vi "Start.vi"(8 "error in (no error)":errorcluster, 11 "Framework in":refnum<class "Framework.lvclass">) -> (0 "error out":errorcluster, 3 "Framework out":refnum<class "Framework.lvclass">)   [LabVIEW 2019, in "DSF Core.lvlib" / "Framework.lvclass"]
uses:
  Framework.lvclass
  Framework States.ctl
  Framework.lvclass/Framework.ctl
  <vilib>/NI/Memory Manager/Classes/Pointer/Pointer.lvclass/Pointer.ctl
  Interface/Interface.lvclass/Interface.ctl
  Pointers/Error/Error Pointer.lvclass/Error Pointer.ctl
  Interface/Dispatcher/Write.vi
  Interface/Dispatcher/Write Dispatcher Command.vi
  Interface/Errors.vi
  Interface/Dispatcher/Invalid Response.vi
  Interface/Dispatcher/Read.vi
  Interface/Dispatcher/Read Dispatcher Response.vi
  Interface/Logging/Send.vi
  Interface/Logging/Send Logging Command.vi
  Interface/Logging/Wait For.vi
  Interface/Logging/Wait For Logging Response.vi
  <vilib>/NI/Memory Manager/Classes/Pointer/Write.vi
  <vilib>/NI/Memory Manager/Classes/Pointer/Write U8.vi
  Read State.vi
  Pointers/Error/Write Error Pointer.vi
  <vilib>/NI/Memory Manager/Classes/Pointer/Get Address.vi
  Interface/Send Command.vi
  Interface/Dispatcher/Command Timeout.vi
  Interface/Dispatcher/Class Name.vi
  <vilib>/NI/Memory Manager/VIs/Write String to Source.vi
  Interface/New Interface Error.vi
  Interface/Wait For Response.vi
  Interface/Dispatcher/Response Timeout.vi
  <vilib>/NI/Memory Manager/Classes/Pointer/Write (No Check).vi
  <vilib>/NI/Memory Manager/Classes/Pointer/Write (No Check) U8.vi
  <vilib>/NI/Memory Manager/Classes/Pointer/Check Move.vi
  <vilib>/NI/Memory Manager/Classes/Pointer/Read.vi
  <vilib>/NI/Memory Manager/Classes/Pointer/Read U8.vi
  <vilib>/NI/Memory Manager/Classes/Pointer/Write 1D U8.vi
  <vilib>/NI/Memory Manager/Classes/Pointer/Clear.vi
  Pointers/Error/Get Power Of 2.vi
  Interface/Write RT FIFO.vi
  <vilib>/NI/Memory Manager/VIs/New Error Cluster.vi
  <vilib>/NI/Memory Manager/VIs/New Error Cluster (512B).vi
  <vilib>/NI/Memory Manager/VIs/Set Error Code.vi
  <vilib>/NI/Memory Manager/VIs/Set Error Status.vi
  <vilib>/NI/Memory Manager/VIs/Set Error Source.vi
  Interface/Interface Error Info.vi
  Interface/Read RT FIFO.vi
  <vilib>/NI/Memory Manager/Classes/Pointer/Check Null Pointer.vi
  <vilib>/NI/Memory Manager/Classes/Pointer/Check Count.vi
  <vilib>/NI/Memory Manager/Classes/Pointer/Check Bounds (Power of 2).vi
  <vilib>/NI/Memory Manager/Classes/Pointer/Read (No Check).vi
  <vilib>/NI/Memory Manager/Classes/Pointer/Read (No Check) U8.vi
  <vilib>/NI/Memory Manager/Classes/Pointer/Write (No Check) 1D U8.vi
  <vilib>/NI/Memory Manager/Classes/Pointer/Clear (No Check).vi
  <vilib>/NI/Memory Manager/Classes/Pointer/Check Length.vi
  VIs/Constants/Constants.vi
  VIs/Constants/Base Error Code.vi
  Interface/Interface Error Offset.vi
  <vilib>/NI/Memory Manager/Classes/Pointer/Errors.vi
  <vilib>/NI/Memory Manager/Classes/Pointer/Null Pointer.vi
  <vilib>/NI/Memory Manager/Classes/Pointer/Is Null.vi
  <vilib>/NI/Memory Manager/Classes/Pointer/Get Size.vi
  <vilib>/NI/Memory Manager/Classes/Pointer/Out of Bounds.vi
  <vilib>/NI/Memory Manager/Classes/Pointer/Check Bounds.vi
  <vilib>/NI/Memory Manager/Classes/Pointer/Check Bounds (Pointer).vi
  <vilib>/NI/Memory Manager/Classes/Pointer/Create Error.vi
  <vilib>/NI/Memory Manager/Classes/Pointer/Write Pointer Size to Error.vi
  <vilib>/NI/Memory Manager/VIs/Write Numeric to Source.vi
  <vilib>/NI/Memory Manager/VIs/Write Numeric Scalar to Source (Base10 U64).vi
  <vilib>/NI/Memory Manager/Classes/Pointer/Check Bounds (Buffer).vi
  <vilib>/NI/Memory Manager/Constants/Constants.vi
  <vilib>/NI/Memory Manager/Constants/Library Name.vi
  <vilib>/NI/Memory Manager/Classes/Pointer/Pointer Error Info.vi
  <vilib>/NI/Memory Manager/Constants/Pointer Class Name.vi
  <vilib>/NI/Memory Manager/Classes/Pointer/Buffer Underflow.vi
  Interface/Logging/Logging Interface.lvclass
  C:/Dev/GitHub/niveristand-data-sharing-framework-custom-device/Core/Classes/Interface/Interface.lvclass
  Interface/Dispatcher/Dispatcher Interface.lvclass
  Pointers/Error/Error Pointer.lvclass
  C:/Program Files (x86)/National Instruments/LabVIEW 2019/vi.lib/NI/Memory Manager/Classes/Pointer/Pointer.lvclass
  VIs/VI Name.vi
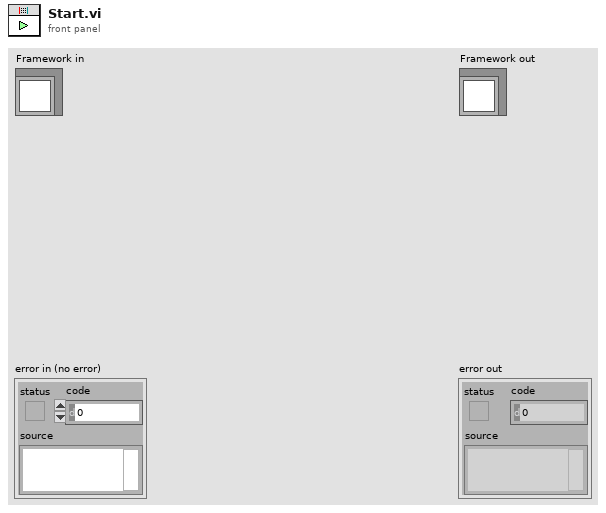
[diagram p1: front panel]
types:
  T1 = typedef "DSF Core.lvlib/Framework.lvclass/Framework States.ctl" = enum8{"Uninitialized", "Initialized", "Start", "Rx", "Tx", "Shutdown"}
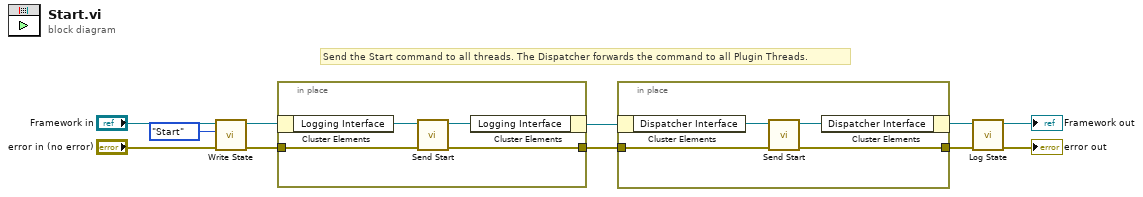
[diagram p0: block diagram]
diagram:
  # "Send the Start command to all threads. The Dispatcher forwards the command to all Plugin Threads."
  n1 = call "Write State.vi"("error in (no error)"="error in (no error)", "state"=Framework_States."Start", "Framework in"="Framework in") -> ("error out"=w8:errorcluster, "Framework out"=w7:refnum<class "Framework.lvclass">)  [unwired: 7 in]
  n2 = in-place {
    in-place-border: w8 -> [w15]
    in-place-border: [w14] -> w11
    n3 = in-place-cluster #1(w7) -> ("Logging Interface"=w13:refnum<class "Logging Interface.lvclass">)
    n4 = call "Send Start.vi"("error in (no error)"=w15, "Logging Interface in"=w13) -> ("error out"=w14:errorcluster, "Logging Interface out"=w12:refnum<class "Logging Interface.lvclass">)  [unwired: 8 in]
    n5 = in-place-cluster #1("Logging Interface"=w12) -> (w10:refnum<class "Framework.lvclass">)
  }
  n6 = in-place {
    in-place-border: w11 -> [w18]
    in-place-border: [w17] -> w3
    n7 = in-place-cluster #2(w10) -> ("Dispatcher Interface"=w19:refnum<class "Dispatcher Interface.lvclass">)
    n8 = call "Send Start.vi"("error in (no error)"=w18, "Dispatcher Interface in"=w19) -> ("error out"=w17:errorcluster, "Dispatcher Interface out"=w16:refnum<class "Dispatcher Interface.lvclass">)  [unwired: 8 in]
    n9 = in-place-cluster #2("Dispatcher Interface"=w16) -> (w4:refnum<class "Framework.lvclass">)
  }
  n10 = call "Log State.vi"("error in (no error)"=w3, "Framework in"=w4) -> ("error out"=→"error out":errorcluster, "Framework out"=→"Framework out":refnum<class "Framework.lvclass">)  [unwired: 8 in]
